vi "Progress Window.vi"(9 "Stop":refnum<data-value>, 10 "Progress":refnum<data-value>, 11 "Status String":refnum<data-value>) -> ()   [LabVIEW 2020, in "Build Automation.lvlib"]
uses:
  Build Automation.lvlib
panel:
  out "Status Message":string
  out "Progress":dbl(slide) scale=0.0..1.0 scale format="%.1f"
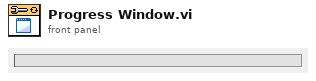
[diagram p1: front panel]
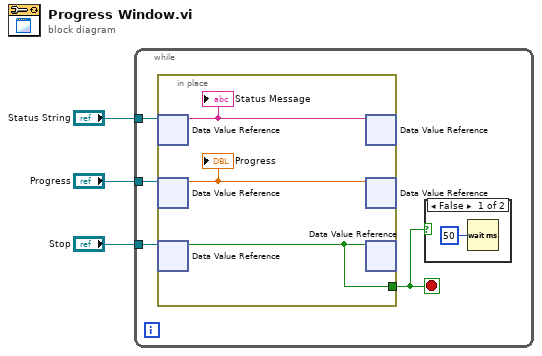
[diagram p0: block diagram]
diagram:
  n1 = while {
    tunnel: "Status String" -> [w7]
    tunnel: "Stop" -> [w6]
    tunnel: "Progress" -> [w5]
    stop <- w4 stop-if-true
    n2 = in-place {
      in-place-border: [w10] -> w4
      n3 = in-place-dvr #1(w7) -> (w11:string)  [unwired: 1 out]
      "Status Message" <- w11
      n4 = in-place-dvr #2(w5) -> (w9:dbl)  [unwired: 1 out]
      "Progress" <- w9
      n5 = in-place-dvr #3(w6) -> (w10:bool)  [unwired: 1 out]
      n6 = in-place-dvr #1(w11) -> ()  [unwired: 2 out]
      n7 = in-place-dvr #2(w9) -> ()  [unwired: 2 out]
      n8 = in-place-dvr #3(w10) -> ()  [unwired: 2 out]
    }
    n9 = case shown="False" w4 {
      frame False {
        n10 = Wait (ms)(milliseconds to wait=u32 50) -> ()  [unwired: 1 out]
      }
      frame True {
      }
    }
  }
